vi "Hypo-T.vi"() -> ()   [LabVIEW 2010]
uses:
  4-High Neurons/4.1.2-Act Neuron TD.ctl
  5.0-Global.vi
  <vilib>/robotics/Obstacle Avoidance/Advanced Vector Field Histogram/NI_Robotics_Vector Field Histogram.lvlib
panel:
  out "XY Graph":cluster{dbl[], sgl[]}(graph)
  out "error out":errorcluster
  out "chosen heading (rad)":dbl
  in  "heading (Degrees)":T1
  out "Heartbeat":bool
  out "Dont Run!":bool
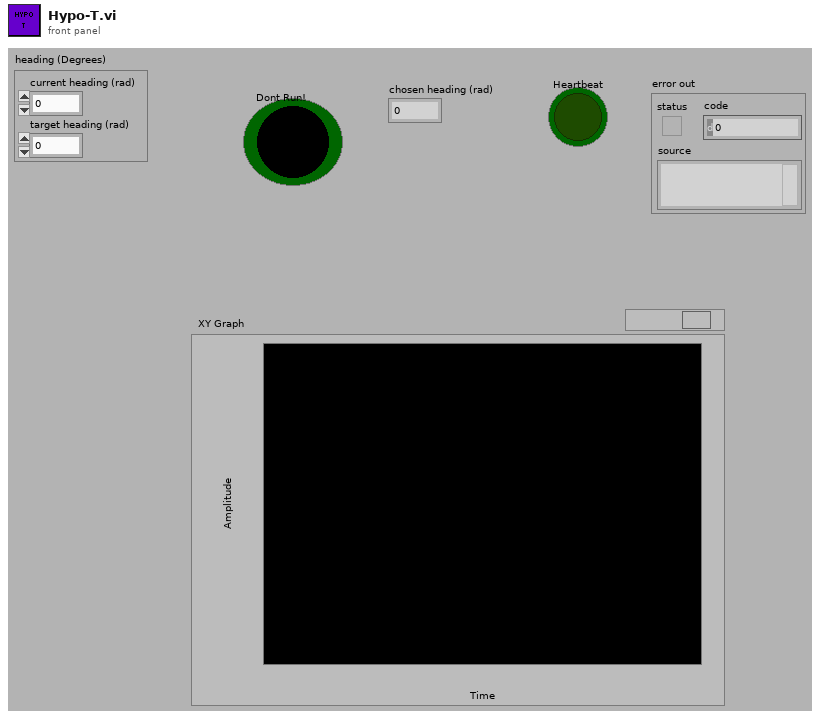
[diagram p1: front panel]
types:
  T1 = cluster{"current heading (rad)":dbl, "target heading (rad)":dbl}
  T2 = typedef "4.1.2-Act Neuron TD.ctl" = cluster{"Speed By Path":sgl[]}
  T3 = cluster{"inner threshold distance":dbl, "outer threshold distance":dbl}
  T4 = enum16{"Set Midbrain Act Data", "Set Forebrain Act Data", "Read Act Data"}
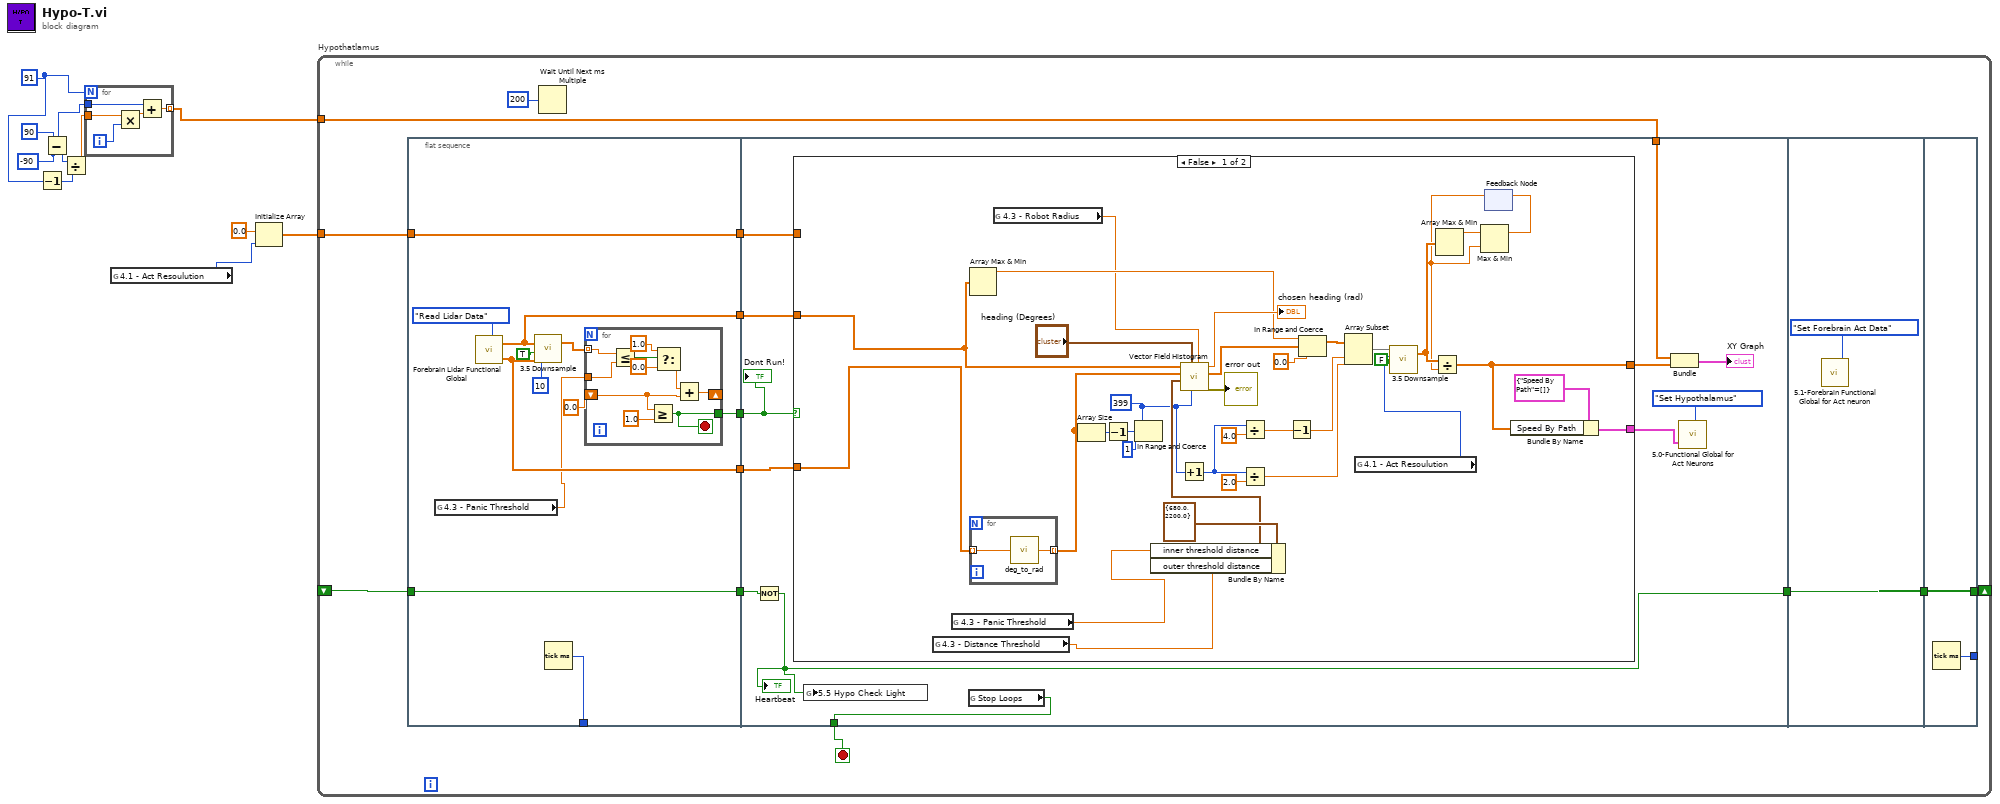
[diagram p0: block diagram]
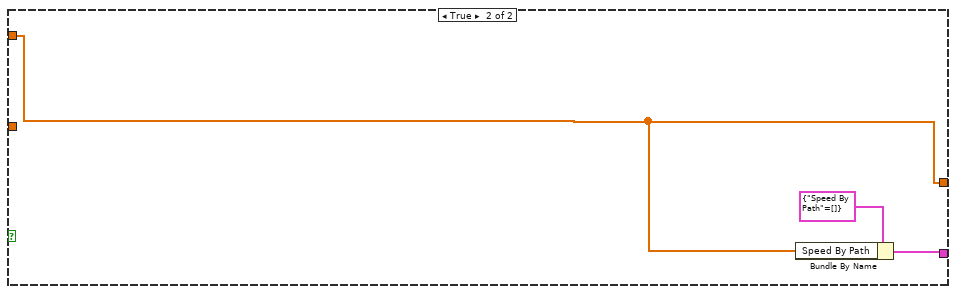
[diagram p2: hidden frame]
diagram:
  w4 = -90
  w3 = 91 ("samples")
  n1 = Decrement(x=w3) -> (x-1=w1:i32)
  n2 = Subtract(x=90, y=w4) -> (x-y=w7:i32)
  n3 = Divide(x=w7, y=w1) -> (x/y=w6:dbl)
  n4 = for {
    N: w3 -> [_]
    tunnel: w6 -> [w14]
    tunnel: w4 -> [w12]
    tunnel: [w11] -> w2 mode=indexing
    i -> [w15]
    n5 = Multiply(x=w14, y=w15) -> (x*y=w13:dbl)
    n6 = Add(x=w12, y=w13) -> (x+y=w11:dbl)
  }
  n7 = global read "5.0-Global.vi" "4.1 - Act Resoulution"() -> (w8:u32)
  n8 = Initialize Array(sgl 0.0 ("element"), w8) -> (w9:sgl[])
  n9 = while "Hypothatlamus" {
    shift-right: [w27] -> _
    shift-left: _ -> [w28]
    tunnel: w9 -> [w21]
    tunnel: w2 -> [w18]
    stop <- w19 stop-if-true
    n10 = flat-sequence {
      tunnel: w28 -> [w40]
      tunnel: [w40] -> w26
      tunnel: [w39] -> _
      tunnel: [w35] -> w24
      tunnel: [w30] -> w23
      tunnel: [w32] -> w22
      tunnel: w21 -> [w31]
      tunnel: [w31] -> w20
      tunnel: w26 -> [w62]
      tunnel: [w57] -> w17
      tunnel: w24 -> [w61]
      tunnel: w23 -> [w60]
      tunnel: w22 -> [w58]
      tunnel: w20 -> [w59]
      tunnel: [w56] -> w19
      tunnel: w18 -> [w55]
      tunnel: w17 -> [w104]
      tunnel: [w104] -> w16
      tunnel: [w106] -> w27
      tunnel: w16 -> [w106]
      tunnel: [w105] -> _
      frame #0 {
        n11 = global read "5.0-Global.vi" "4.3 - Panic Threshold"() -> (w29:dbl)
        n12 = call "Forebrain Lidar Functional Global.vi"("Lidar Action"=enum16{"Set Lidar Data", "Read Lidar Data"}."Read Lidar Data") -> ("Lidar Angle Data Out (Degrees)"=w30:sgl[], "Lidar Magnitude Data Out (mm)"=w35:sgl[])  [unwired: 2 in]
        n13 = call "3.5 Downsample.vi"("Corresponding Input Array For Minimum"=w30, "Minimum?"=TRUE, "Numeric"=10, "Input Array"=w35) -> ("Output Array"=w34:sgl[])  [unwired: 1 out]
        n14 = Tick Count (ms)() -> (millisecond timer value=w39:u32)
        n15 = for {
          shift-right: [w44] -> _
          shift-left: 0.0 -> [w43]
          tunnel: w34 -> [w50] mode=indexing
          tunnel: w29 -> [w49]
          tunnel: [w41] -> w32
          stop <- w41 stop-if-true
          n16 = Less Or Equal?(x=w50, y=w49) -> (x <= y?=w48:bool)
          n17 = Greater Or Equal?(x=w43, y=1.0) -> (x >= y?=w41:bool)
          n18 = Select(t=1.0, s=w48, f=0.0) -> (s? t:f=w45:dbl)
          n19 = Add(x=w45, y=w43) -> (x+y=w44:dbl)
        }
      }
      frame #1 {
        n20 = Not(x=w62) -> (.not. x?=w57:bool)
        "Heartbeat" <- w57
        n21 = case shown="False" w58 {
          tunnel: [w64 w101] -> w54
          tunnel: w61 -> [w71 _]
          tunnel: w60 -> [w70 _]
          tunnel: w59 -> [_ w101]
          tunnel: [w63 w100] -> w52
          frame False {
            w73 = 399 ("# bins")
            n22 = global read "5.0-Global.vi" "4.3 - Distance Threshold"() -> (w68:dbl)
            n23 = global read "5.0-Global.vi" "4.3 - Panic Threshold"() -> (w67:dbl)
            n24 = Array Max & Min(array=w71) -> (max value=w91:sgl)  [unwired: 3 out]
            n25 = for {
              tunnel: w70 -> [w99] mode=indexing
              tunnel: [w98] -> w77 mode=indexing
              n26 = call "deg_to_rad.vi"("Degrees"=w99) -> ("Radians"=w98:dbl)
            }
            n27 = global read "5.0-Global.vi" "4.3 - Robot Radius"() -> (w66:dbl)
            n28 = Array Size(array=w77) -> (size(s)=w76:i32)
            n29 = Decrement(x=w76) -> (x-1=w74:i32)
            n30 = In Range and Coerce(upper limit=w73, x=w74, lower limit=1) -> ()  [unwired: 2 out]
            n31 = Bundle By Name(cluster=T3 {"inner threshold distance"=680.0, "outer threshold distance"=2200.0} ("thresholds"), "inner threshold distance"=w67, "outer threshold distance"=w68) -> (w78:T3)
            n32 = call <vilib>:"Vector Field Histogram.vi"("obstacle clearance distance"=w66, "# bins"=w73, "heading"="heading (Degrees)", "thresholds"=w78, "direction angles (rad)"=w77, "distances"=w71) -> ("error out"=→"error out":errorcluster, "histogram"=w81:dbl[], "chosen heading (rad)"=→"chosen heading (rad)":dbl)  [unwired: 2 in, 1 out]
            n33 = Increment(x=w73) -> (x+1=w82:i32)
            n34 = Divide(x=w82, y=4.0) -> (x/y=w87:dbl)
            n35 = Divide(x=w82, y=2.0) -> (x/y=w84:dbl)
            n36 = Decrement(x=w87) -> (x-1=w86:dbl)
            n37 = In Range and Coerce(upper limit=w91, x=w81, lower limit=0.0 ("obstacle clearance distance")) -> (coerced(x)=w80:dbl[])  [unwired: 1 out]
            n38 = Array Subset(array=w80, index=w86, length=w84) -> (w83:dbl[])
            n39 = global read "5.0-Global.vi" "4.1 - Act Resoulution"() -> (w69:u32)
            n40 = call "3.5 Downsample.vi"("Minimum?"=FALSE, "Numeric"=w69, "Input Array"=w83) -> ("Output Array"=w92:sgl[])  [unwired: 1 in, 1 out]
            n41 = Array Max & Min(array=w92) -> (max value=w96:sgl)  [unwired: 3 out]
            n42 = feedback #1() -> (w89:sgl)  [unwired: 1 in]
            n43 = Divide(x=w92, y=w89) -> (x/y=w64:sgl[])
            n44 = Max & Min(x=w96, y=w89) -> (max(x,y)=w95:sgl)  [unwired: 1 out]
            n45 = feedback-in #1(w95) -> ()
            n46 = Bundle By Name(cluster=T2 {"Speed By Path"=[]} ("Forebrain Act Neurons"), "Speed By Path"=w64) -> (w63:T2)
          }
          frame True {
            n47 = Bundle By Name(cluster=T2 {"Speed By Path"=[]} ("Forebrain Act Neurons"), "Speed By Path"=w101) -> (w100:T2)
          }
        }
        n48 = global write "5.0-Global.vi" "5.5 Hypo Check Light"(w57) -> ()
        n49 = global read "5.0-Global.vi" "Stop Loops"() -> (w56:bool)
        n50 = Bundle(w55, w54) -> (→"XY Graph":cluster{dbl[], sgl[]})  [unwired: 1 in]
        n51 = call "5.0-Functional Global for Act Neurons.vi"("Input Act Neurons"=w52, "Mode"=enum16{"Set Hypothalamus", "Read Hypothalamus"}."Set Hypothalamus") -> ()  [unwired: 1 out]
        "Dont Run!" <- w58
      }
      frame #2 {
        n52 = call "5.1-Forebrain Functional Global for Act neuron.vi"("Command"=T4."Set Forebrain Act Data") -> ()  [unwired: 1 in, 1 out]
      }
      frame #3 {
        n53 = Tick Count (ms)() -> (millisecond timer value=w105:u32)
      }
    }
    n54 = Wait Until Next ms Multiple(millisecond multiple=u32 200) -> ()  [unwired: 1 out]
  }
